vi "Simple demo.vi"() -> ()   [LabVIEW 2021]
uses:
  Z:/Samples/LabVIEW/Library/UnderAutomation.UniversalRobots.dll
  Library/UnderAutomation.UniversalRobots.dll
panel:
  out "Powered on":bool
  in  "Script to execute":string
  in  "Send script":bool
  out "Z":dbl
  out "Y":dbl
  out "X":dbl
  in  "Robot IP":string
  out "Connect error":errorcluster
  in  "Power off":bool
  in  "Power on\nRelease brake":bool
  out "Connected":bool
  out "License state":string
  in  "Connect":bool
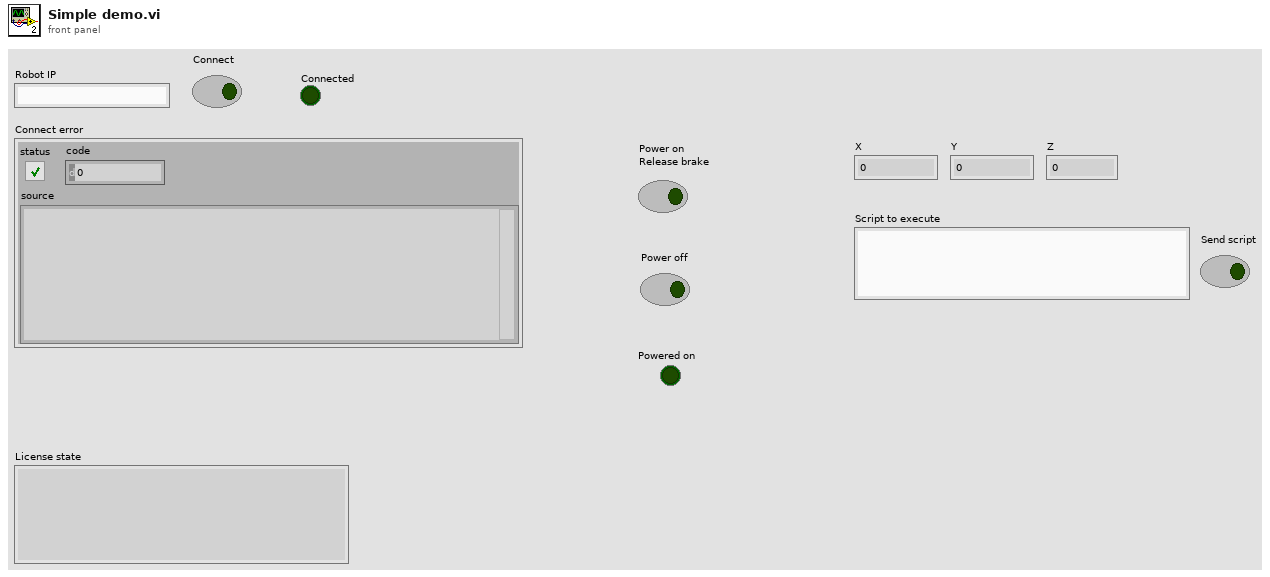
[diagram p1: front panel]
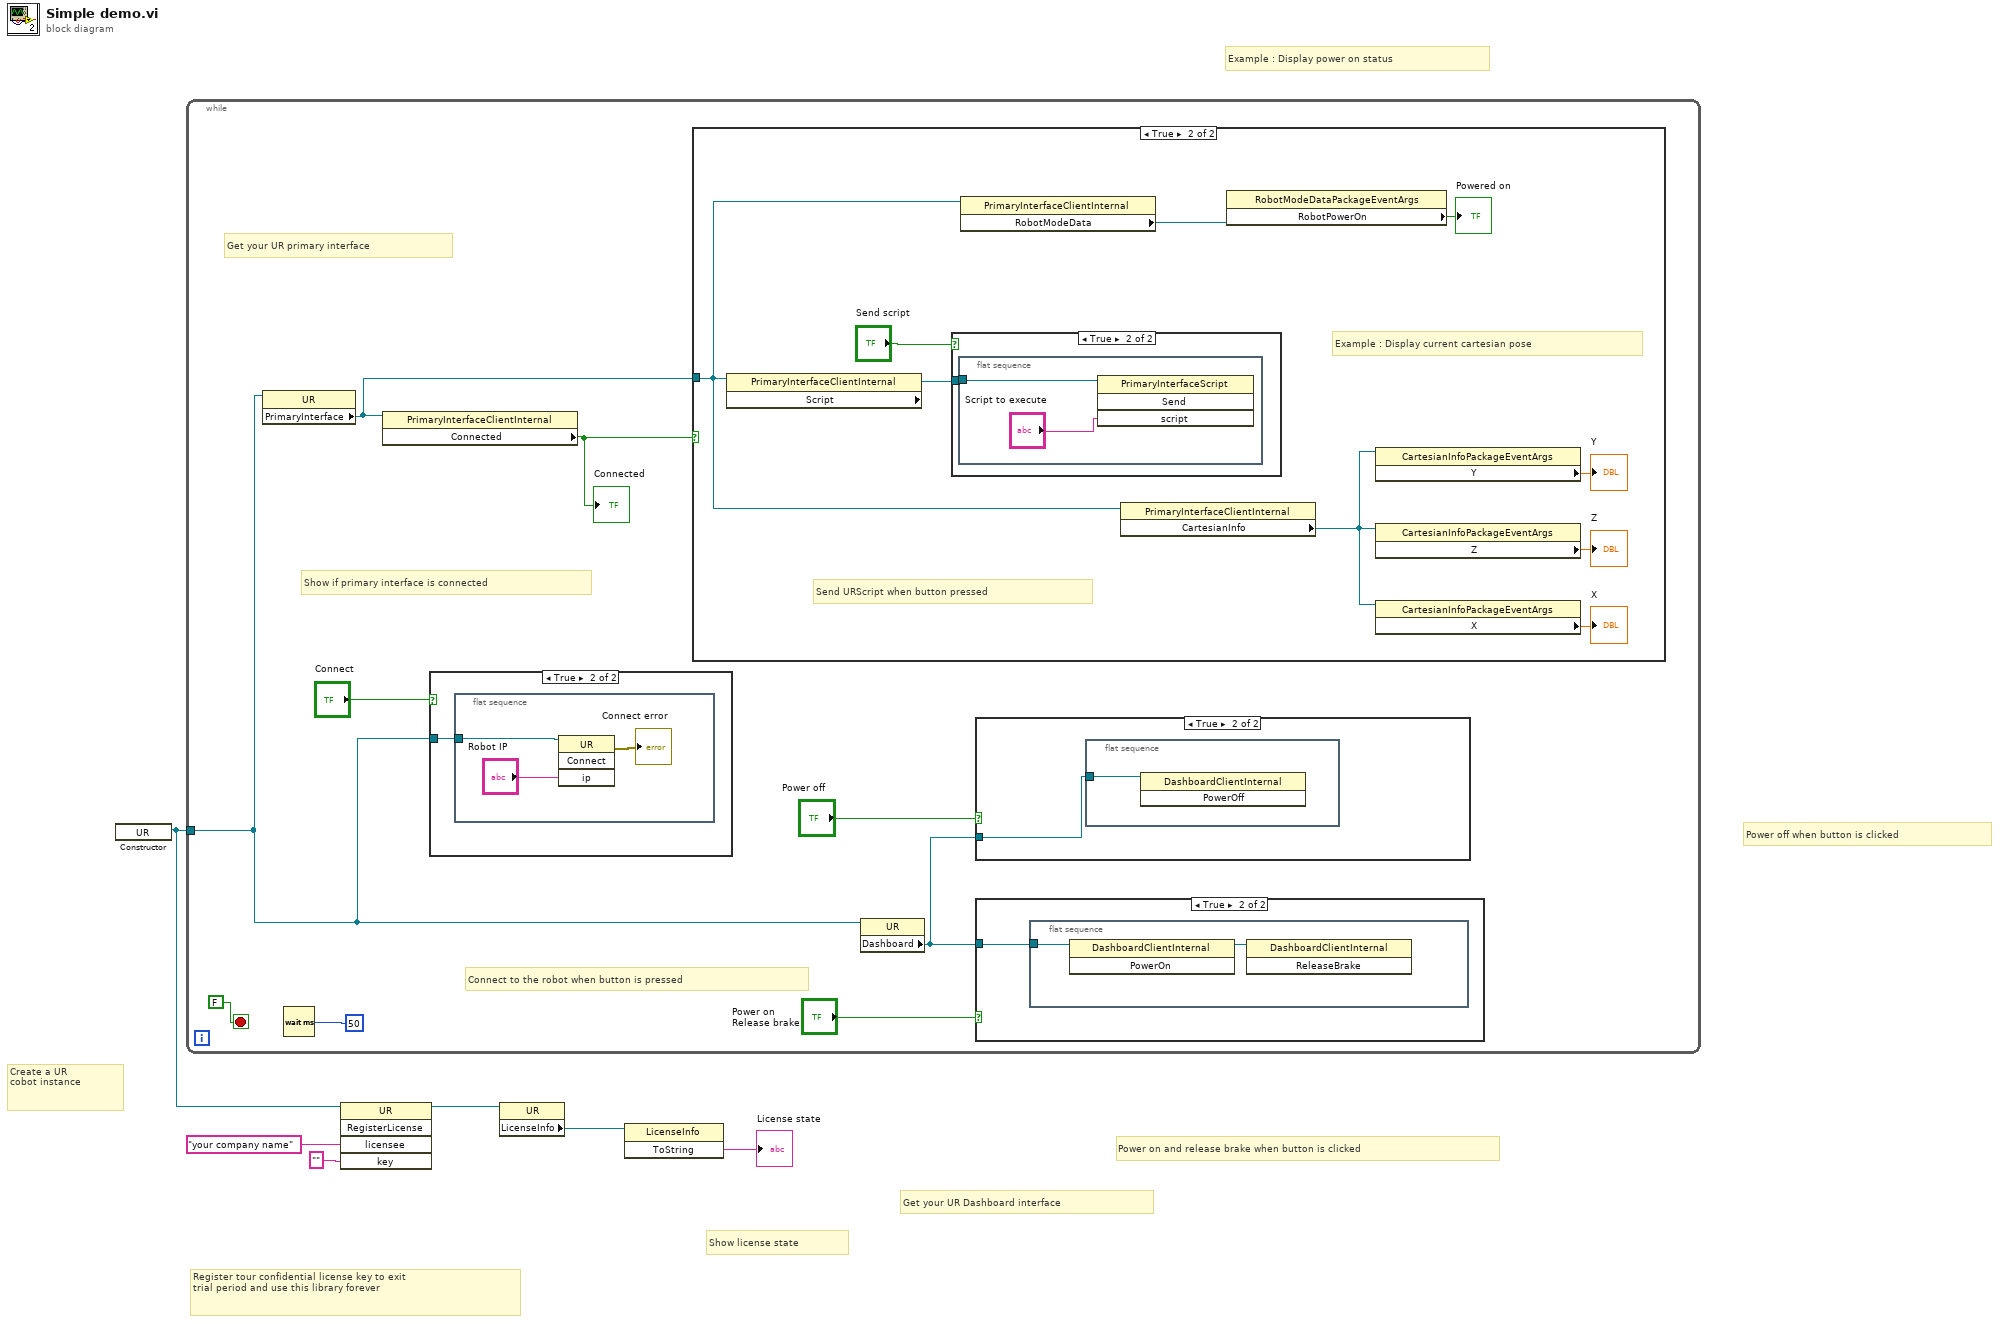
[diagram p0: block diagram]
diagram:
  # "Example : Display power on status"
  # "Create a UR\ncobot instance"
  # "Show license state"
  # "Register tour confidential license key to exit\ntrial period and use this library forever"
  # "Power off when button is clicked"
  # "Power on and release brake when button is clicked"
  # "Get your UR Dashboard interface"
  n1 = constructor class="UR"() -> (reference out=w1:refnum<k24>)  [unwired: 3 in, 2 out]
  n2 = while {
    tunnel: w1 -> [w10]
    stop <- FALSE stop-if-true
    # "Connect to the robot when button is pressed"
    # "Show if primary interface is connected"
    # "Get your UR primary interface"
    n3 = property class="UR"(reference=w10) -> ("PrimaryInterface"=w9:refnum<k24>)  [unwired: 1 in, 2 out]
    n4 = Wait (ms)(milliseconds to wait=u32 50) -> ()  [unwired: 1 out]
    n5 = property class="PrimaryInterfaceClientInternal"(reference=w9) -> ("Connected"=w8:bool)  [unwired: 1 in, 2 out]
    "Connected" <- w8
    n6 = case shown="True" "Connect" {
      tunnel: w10 -> [_ w33]
      frame False {
      }
      frame True {
        n7 = flat-sequence {
          tunnel: w33 -> [w35]
          frame #0 {
            n8 = invoke class="UR" method="Connect"(reference=w35, "ip"="Robot IP") -> (error out=→"Connect error":errorcluster)  [unwired: 2 in, 3 out]
          }
        }
      }
    }
    n9 = case shown="True" w8 {
      tunnel: w9 -> [_ w16]
      frame False {
      }
      frame True {
        # "Send URScript when button pressed"
        # "Example : Display current cartesian pose"
        n10 = property class="PrimaryInterfaceClientInternal"(reference=w16) -> ("Script"=w23:refnum<k24>)  [unwired: 1 in, 2 out]
        n11 = case shown="True" "Send script" {
          tunnel: w23 -> [_ w25]
          frame False {
          }
          frame True {
            n12 = flat-sequence {
              tunnel: w25 -> [w27]
              frame #0 {
                n13 = invoke class="PrimaryInterfaceScript" method="Send"(reference=w27, "script"="Script to execute") -> ()  [unwired: 2 in, 4 out]
              }
            }
          }
        }
        n14 = property class="PrimaryInterfaceClientInternal"(reference=w16) -> ("RobotModeData"=w22:refnum<k24>)  [unwired: 1 in, 2 out]
        n15 = property class="PrimaryInterfaceClientInternal"(reference=w16) -> ("CartesianInfo"=w17:refnum<k24>)  [unwired: 1 in, 2 out]
        n16 = property class="RobotModeDataPackageEventArgs"(reference=w22) -> ("RobotPowerOn"=→"Powered on":bool)  [unwired: 1 in, 2 out]
        n17 = property class="CartesianInfoPackageEventArgs"(reference=w17) -> ("Y"=→"Y":dbl)  [unwired: 1 in, 2 out]
        n18 = property class="CartesianInfoPackageEventArgs"(reference=w17) -> ("Z"=→"Z":dbl)  [unwired: 1 in, 2 out]
        n19 = property class="CartesianInfoPackageEventArgs"(reference=w17) -> ("X"=→"X":dbl)  [unwired: 1 in, 2 out]
      }
    }
    n20 = property class="UR"(reference=w10) -> ("Dashboard"=w11:refnum<k24>)  [unwired: 1 in, 2 out]
    n21 = case shown="True" "Power off" {
      tunnel: w11 -> [_ w28]
      frame False {
      }
      frame True {
        n22 = flat-sequence {
          tunnel: w28 -> [w29]
          frame #0 {
            n23 = invoke class="DashboardClientInternal" method="PowerOff"(reference=w29) -> ()  [unwired: 2 in, 3 out]
          }
        }
      }
    }
    n24 = case shown="True" "Power on\nRelease brake" {
      tunnel: w11 -> [_ w30]
      frame False {
      }
      frame True {
        n25 = flat-sequence {
          tunnel: w30 -> [w32]
          frame #0 {
            n26 = invoke class="DashboardClientInternal" method="PowerOn"(reference=w32) -> (reference out=w31:refnum<k24>)  [unwired: 2 in, 2 out]
            n27 = invoke class="DashboardClientInternal" method="ReleaseBrake"(reference=w31) -> ()  [unwired: 2 in, 3 out]
          }
        }
      }
    }
  }
  n28 = invoke class="UR" method="RegisterLicense"(reference=w1, "licensee"="your company name", "key"="") -> (reference out=w3:refnum<k24>)  [unwired: 2 in, 4 out]
  n29 = property class="UR"(reference=w3) -> ("LicenseInfo"=w2:refnum<k24>)  [unwired: 1 in, 2 out]
  n30 = invoke class="LicenseInfo" method="ToString"(reference=w2) -> ("ToString"=→"License state":string)  [unwired: 2 in, 2 out]
